vi "BRig_RT_genNoise_AnaIn.vi"() -> (1 "AI_1":i16, 2 "AI_0":i16)   [LabVIEW 2014]
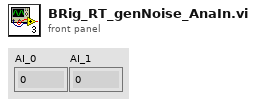
[diagram p1: front panel]
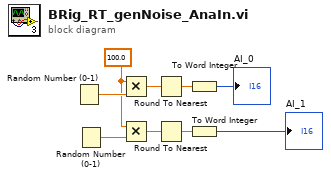
[diagram p0: block diagram]
diagram:
  w7 = 100.0 ("x")
  n1 = Random Number (0-1)() -> (number: 0 to 1=w9:dbl)
  n2 = Random Number (0-1)() -> (number: 0 to 1=w8:dbl)
  n3 = Multiply(x=w7, y=w9) -> (x*y=w6:dbl)
  n4 = Multiply(x=w7, y=w8) -> (x*y=w5:dbl)
  n5 = Round To Nearest(number=w6) -> (nearest integer value=w4:dbl)
  n6 = Round To Nearest(number=w5) -> (nearest integer value=w3:dbl)
  n7 = To Word Integer(number=w4) -> (16bit integer=→"AI_0":i16)
  n8 = To Word Integer(number=w3) -> (16bit integer=→"AI_1":i16)
